vi "FormatCommand.vi"(11 "Command":string) -> (3 "Formatted Command":string)   [LabVIEW 2012, in "Omega-CSi32.lvlib"]
uses:
  Omega-CSi32.lvlib
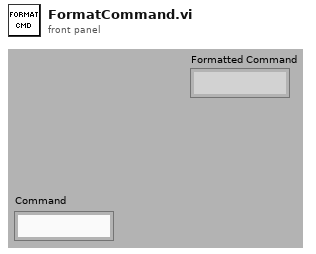
[diagram p1: front panel]
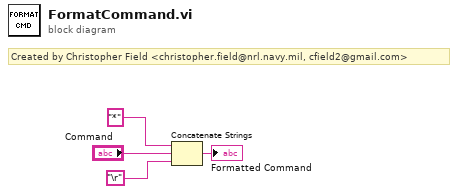
[diagram p0: block diagram]
diagram:
  # "Created by Christopher Field <christopher.field@nrl.navy.mil, cfield2@gmail.com>"
  n1 = Concatenate Strings("*", "Command", "\r") -> (→"Formatted Command":string)
